vi "Добавить точку на рисунок (SubVI).vi"(0 "in picture":picture, 1 "dot х":u16 step=1, 2 "dot y":u16 step=1, 3 "thickness":u16 step=1, 4 "цвет":u32(colorbox), 5 "error in":errorcluster) -> (14 "out picture":picture, 19 "error out":errorcluster)   [LabVIEW 2013]
panel:
  in  "Style":T1(ring)
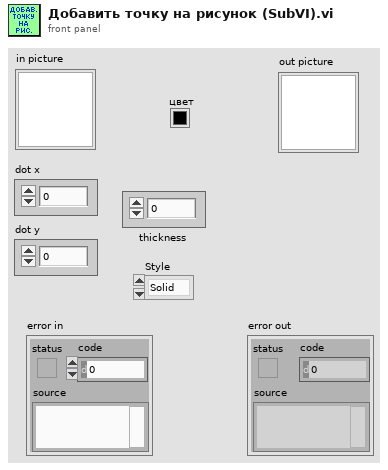
[diagram p1: front panel]
types:
  T1 = enum32{"Solid", "Dash", "Dot", "DashDot", "DashDotDot"}
  T2 = cluster{"thickness":u16, "Style":enum32{"Solid", "Dash", "Dot", "DashDot", "DashDotDot"}}
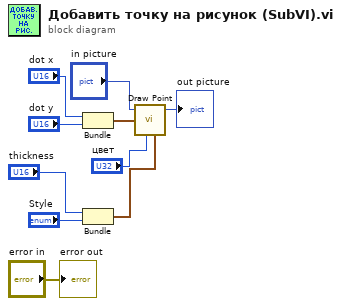
[diagram p0: block diagram]
diagram:
  n1 = Bundle("dot х"="dot х", "dot y"="dot y") -> (w6:cluster{"dot х":u16, "dot y":u16})  [unwired: 1 in]
  n2 = Bundle("thickness"="thickness", "Style"="Style") -> (w9:T2)  [unwired: 1 in]
  n3 = call <vilib>:"Draw Point.vi"("picture"="in picture", "point(x,y)"=w6, "color(black)"="цвет", "pen"=w9) -> ("new picture"=→"out picture":picture)  [unwired: 5 in]
  "error out" <- "error in"
